vi "Controller Write BPM or PS Filter Data and Address.vi"(0 "BPM-PS ADDR":refnum<k21>[](array[refnum]), 5 "BPM-PS DATA":refnum<k21>[](array[refnum]), 7 "Address":u16, 9 "Data":fxp<+/-,22,4>[](array[numeric]), 11 "error in":errorcluster) -> (15 "error out":errorcluster)   [LabVIEW 2011, in "Controller VIs.lvlib"]
uses:
  Controller VIs.lvlib
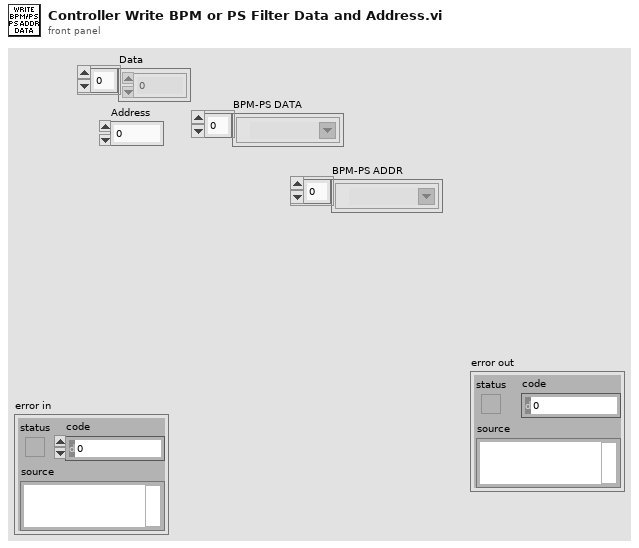
[diagram p1: front panel]
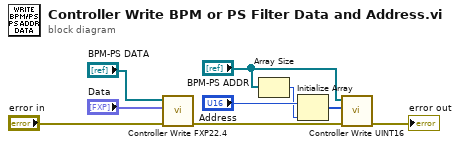
[diagram p0: block diagram]
diagram:
  n1 = call "Controller Write FXP22.4.vi"("Error In"="error in", "Values"="Data", "Variables"="BPM-PS DATA") -> ("Error Out"=w5:errorcluster)  [unwired: 8 in]
  n2 = Array Size(array="BPM-PS ADDR") -> (size(s)=w3:i32)
  n3 = Initialize Array("Address", w3) -> (w6:u16[])
  n4 = call "Controller Write UINT16.vi"("error in (no error)"=w5, "Values"=w6, "Variables"="BPM-PS ADDR") -> ("error out"=→"error out":errorcluster)  [unwired: 8 in]
